vi "Select Query SQLServer.vi"(5 "Order By":string, 7 "Where":string, 8 "error in (no error)":errorcluster, 9 "Column Names":string[](array[string]), 10 "Table Name":string, 11 "ADODB._Connection":refnum<k7>) -> (0 "error out":errorcluster, 1 "element":string, 2 "Selected Data":string[][](array[string]), 3 "ADODB._Connection 2":refnum<k7>)   [LabVIEW 2017]
panel:
  out "Query":string
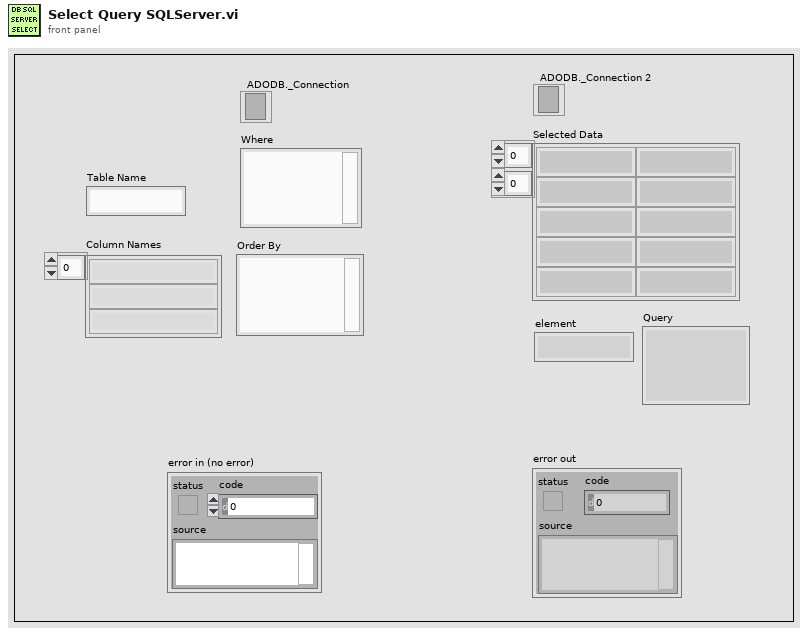
[diagram p1: front panel]
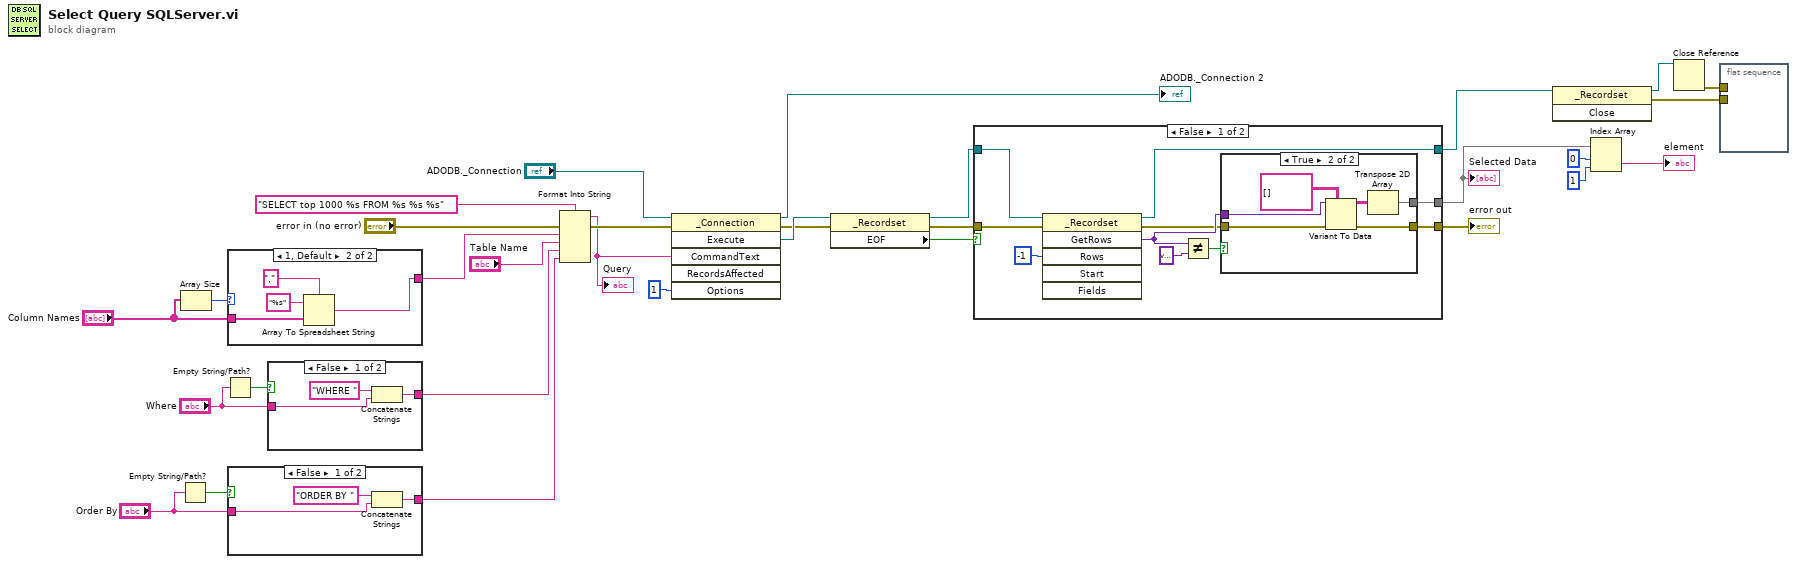
[diagram p0: block diagram]
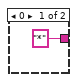
[diagram p2: hidden frame]
diagram:
  n1 = Empty String/Path?(string/path="Order By") -> (empty?=w26:bool)
  n2 = Array Size(array="Column Names") -> (size(s)=w7:i32)
  n3 = Empty String/Path?(string/path="Where") -> (empty?=w30:bool)
  n4 = case shown="1, Default" w7 {
    tunnel: ["*" ("CommandText") w33] -> w2
    tunnel: "Column Names" -> [_ w36]
    frame 0 {
    }
    frame 1, Default {
      n5 = Array To Spreadsheet String(delimiter (Tab)=",", array=w36, 3:"%s" ("format string")) -> (spreadsheet string=w33:string)
    }
  }
  n6 = case shown="False" w26 {
    tunnel: "Order By" -> [w39 _]
    tunnel: [w37 _] -> w4
    frame False {
      n7 = Concatenate Strings("ORDER BY " ("string"), w39) -> (w37:string)
    }
    frame True {
    }
  }
  n8 = case shown="False" w30 {
    tunnel: "Where" -> [w42 _]
    tunnel: [w40 _] -> w5
    frame False {
      n9 = Concatenate Strings("WHERE " ("string"), w42) -> (w40:string)
    }
    frame True {
    }
  }
  n10 = Format Into String(format string="SELECT top 1000 %s FROM %s %s %s" ("CommandText"), error in="error in (no error)", w2, "Table Name", w5, w4) -> (resulting string=w14:string, error out=w28:errorcluster)  [unwired: 1 in]
  "Query" <- w14
  n11 = invoke class="_Connection" method="Execute"(reference="ADODB._Connection", error in=w28, "CommandText"=w14, "Options"=1) -> (reference out=→"ADODB._Connection 2":refnum<k7>, error out=w23:errorcluster, "Execute"=w24:refnum<k7>)  [unwired: 2 in, 3 out]
  n12 = property class="_Recordset"(reference=w24, error in=w23) -> (reference out=w20:refnum<k7>, error out=w22:errorcluster, "EOF"=w21:bool)
  n13 = case shown="False" w21 {
    tunnel: [w52 _] -> w17
    tunnel: [w51 _] -> w12
    tunnel: w20 -> [w46 w60]
    tunnel: w22 -> [w45 _]
    tunnel: [w43 w60] -> w19
    frame False {
      n14 = invoke class="_Recordset" method="GetRows"(reference=w46, error in=w45, "Rows"=-1) -> (reference out=w43:refnum<k7>, error out=w44:errorcluster, "GetRows"=w47:variant)  [unwired: 3 in, 3 out]
      n15 = Not Equal?(x=w47, y=variant) -> (x != y?=w48:bool)
      n16 = case shown="True" w48 {
        tunnel: w47 -> [_ w58]
        tunnel: w44 -> [w53 w59]
        tunnel: [w53 w56] -> w52
        tunnel: [_ w54] -> w51
        frame False {
        }
        frame True {
          n17 = Variant To Data(error in=w59, type=string[][] [], Variant=w58) -> (data=w55:string[][], error out=w56:errorcluster)
          n18 = Transpose 2D Array(2D array=w55) -> (transposed array=w54:string[][])
        }
      }
    }
    frame True {
    }
  }
  "error out" <- w17
  "Selected Data" <- w12
  n19 = invoke class="_Recordset" method="Close"(reference=w19) -> (reference out=w16:refnum<k7>, error out=w18:errorcluster)  [unwired: 2 in, 1 out]
  n20 = Index Array(array=w12, index (row)=0, index (col)=1 ("disabled index (col)")) -> (element=→"element":string)
  n21 = Close Reference(reference=w16) -> (error out=w15:errorcluster)  [unwired: 1 in]
  n22 = flat-sequence {
    tunnel: w18 -> [_]
    tunnel: w15 -> [_]
    frame #0 {
    }
  }
